vi "IntakeNetwork.vi"(8 "error in (no error)":errorcluster) -> (0 "error out":errorcluster)   [LabVIEW 2023]
uses:
  IntakeGlobal.vi
  <vilib>/Rock Robotics/Network Tables/NT Write Number.vi
  <vilib>/Rock Robotics/Network Tables/NT Write Boolean.vi
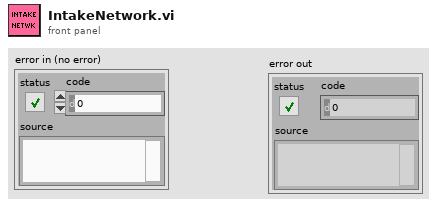
[diagram p1: front panel]
types:
  T1 = typedef "IntakeState.ctl" = enum16{"0-init", "1-cancel", "2-wait-for-cmd", "3-intake-check-for-note", "4-intake-start-intake", "5-intake-have-note-yet", "6-intake-stop-motor", "7-spit-out", "8-feed-note-to-shooter"}
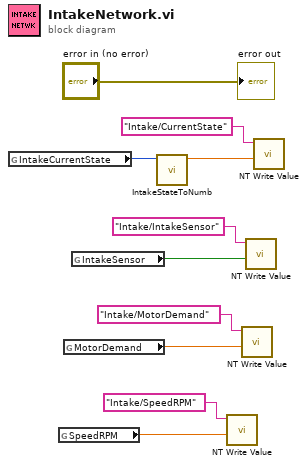
[diagram p0: block diagram]
diagram:
  n1 = global read "IntakeGlobal.vi" "IntakeCurrentState"() -> (w2:T1)
  n2 = global read "IntakeGlobal.vi" "SpeedRPM"() -> (w9:dbl)
  n3 = global read "IntakeGlobal.vi" "MotorDemand"() -> (w4:dbl)
  n4 = global read "IntakeGlobal.vi" "IntakeSensor"() -> (w6:bool)
  n5 = call "IntakeStateToNumb.vi"("Intake_State"=w2) -> ("StateNumber"=w1:dbl)  [unwired: 10 in]
  n6 = call-poly <vilib>:"NT Write Value.vi"("value"=w9, "name"="Intake/SpeedRPM") -> ()  [unwired: 9 in, 1 out]
  n7 = call-poly <vilib>:"NT Write Value.vi"("value"=w4, "name"="Intake/MotorDemand") -> ()  [unwired: 9 in, 1 out]
  n8 = call-poly <vilib>:"NT Write Value.vi"("value"=w6, "name"="Intake/IntakeSensor") -> ()  [unwired: 9 in, 1 out]
  n9 = call-poly <vilib>:"NT Write Value.vi"("value"=w1, "name"="Intake/CurrentState") -> ()  [unwired: 9 in, 1 out]
  "error out" <- "error in (no error)"
